vi "BlinkLED.vi"() -> ()   [LabVIEW 2017]
panel:
  in  "Array":dbl[](array[numeric])
  out "Boolean":bool
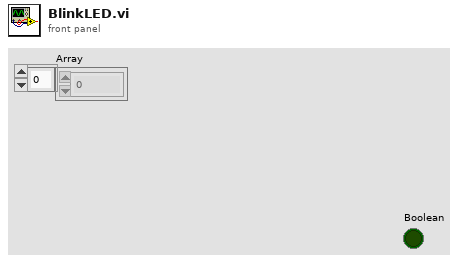
[diagram p1: front panel]
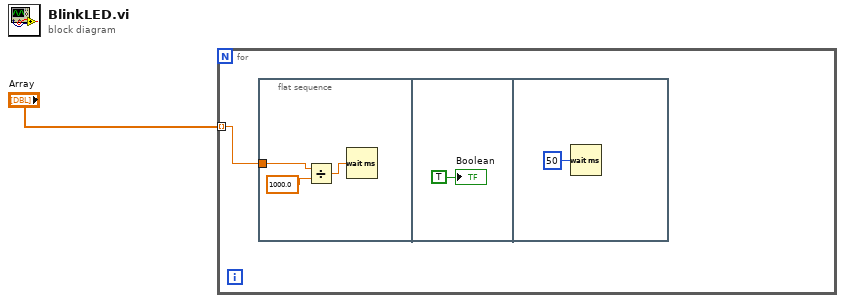
[diagram p0: block diagram]
diagram:
  n1 = for {
    tunnel: "Array" -> [w2] mode=indexing
    n2 = flat-sequence {
      tunnel: w2 -> [w5]
      frame #0 {
        n3 = Divide(x=w5, y=1000.0) -> (x/y=w4:dbl)
        n4 = Wait (ms)(milliseconds to wait=w4) -> ()  [unwired: 1 out]
      }
      frame #1 {
        "Boolean" <- TRUE ("Boolean")
      }
      frame #2 {
        n5 = Wait (ms)(milliseconds to wait=u32 50) -> ()  [unwired: 1 out]
      }
    }
  }
